vi "Player Info.vi"(11 "TeamEffort in":refnum<class "TeamEffort.lvclass">) -> (1 "Victory Speach":string="There is no 'I' in TEAM!", 2 "Name":string="Team Effort!", 3 "TeamEffort out":refnum<class "TeamEffort.lvclass">)   [LabVIEW 2015, in "TeamEffort.lvclass"]
uses:
  TeamEffort.lvclass
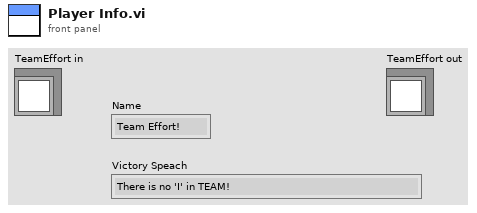
[diagram p1: front panel]
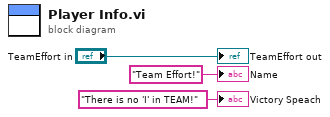
[diagram p0: block diagram]
diagram:
  "TeamEffort out" <- "TeamEffort in"
  "Name" <- "Team Effort!" ("Name")
  "Victory Speach" <- "There is no 'I' in TEAM!" ("Victory Speach")
